vi "IndexArray.vi"() -> ()   [LabVIEW 2021]
panel:
  out "element 2":dbl
  out "element":dbl
  in  "Array":dbl[](array[numeric])
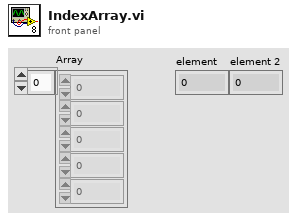
[diagram p1: front panel]
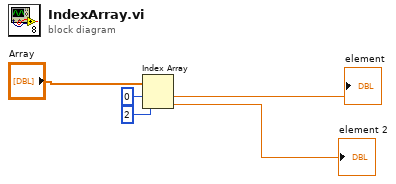
[diagram p0: block diagram]
diagram:
  n1 = Index Array(array="Array", index #1=0 ("index"), index #2=2 ("index")) -> (element #1=→"element":dbl, element #2=→"element 2":dbl)
